vi "Read Image (MMF) (SubVI).vi"(0 "FPGA REF (MWT) IN":T3, 1 "Experiment Mode":T1=enum."Replay", 3 "Image Size":T4 {"Width" step=8; "Height" step=8}, 12 "Frame Number":u64, 13 "TimeStamp":u64) -> (4 "Image Data":T2, 6 "Data Valid?":bool)   [LabVIEW 2020]
uses:
  Controls (HOST)/Image Size.ctl
  Controls (HOST)/FPGA REF (MWT).ctl
  Controls (HOST)/Data to Disk Bundle.ctl
  Controls (HOST)/Experiment Mode.ctl
  <vilib>/Utility/error.llb/Error Cluster From Error Code.vi
  <vilib>/rvi/errors/niLvFpgaAdjustHostInterfaceError.vi
  <vilib>/rvi/interface/nirviMethod/nirviMethod.xnode
  <vilib>/rvi/errors/niLvFpgaMergeErrorWithErrorCode.vi
  <vilib>/FPGAPlugInAG/Dynamic/niLvFpga_AcquireReadRegionFifo_Dynamic.vi
  <vilib>/FPGAPlugInAG/Dynamic/niLvFpga_ReadFifo_Dynamic.vi
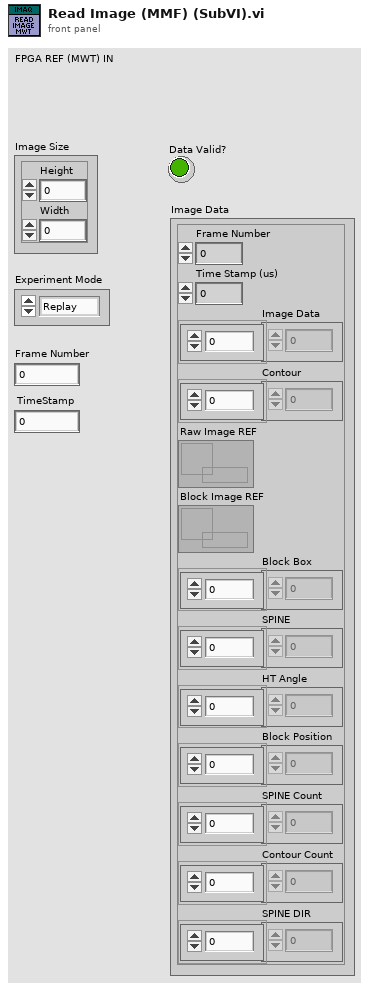
[diagram p1: front panel]
types:
  T1 = typedef "Experiment Mode.ctl" = enum16{"Live", "Replay"}
  T2 = typedef "Data to Disk Bundle.ctl" = cluster{"Frame Number":u64, "Time Stamp (us)":u64, "Image Data":u64[], "Contour":u32[], "Raw Image REF":refnum<data-value>, "Block Image REF":refnum<data-value>, "Block Box":u64[], "SPINE":u32[], "HT Angle":u64[], "Block Position":u64[], "SPINE Count":u32[], "Contour Count":u32[], "SPINE DIR":u8[]}
  T3 = typedef "FPGA REF (MWT).ctl" = refnum<k20>
  T4 = typedef "Image Size.ctl" = cluster{"Height":u16, "Width":u16}
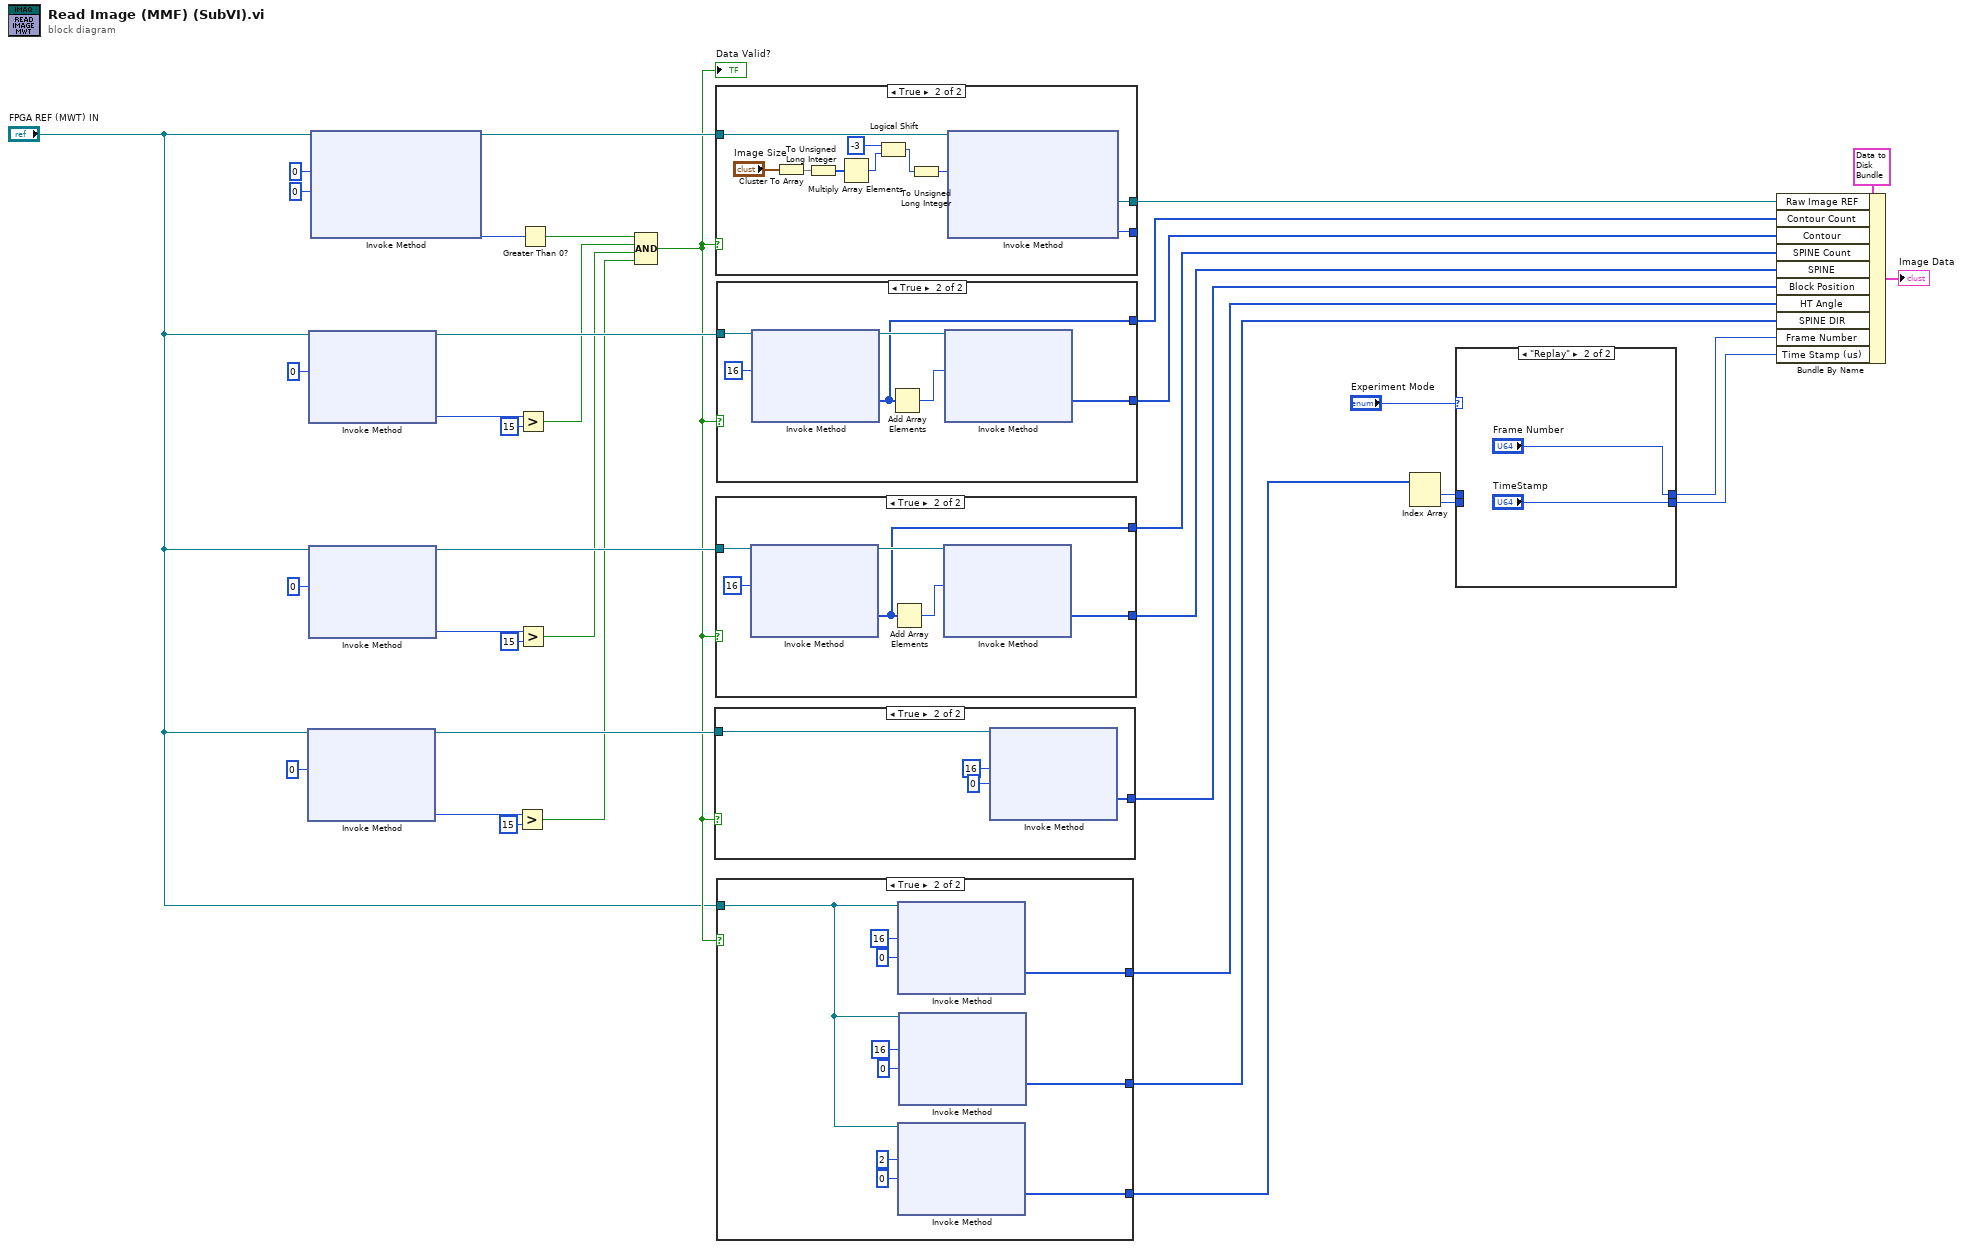
[diagram p0: block diagram]
diagram:
  n1 = xnode "Invoke Method"("FPGA VI Reference In"="FPGA REF (MWT) IN", "Number of Elements"=u32 0) -> ("FPGA VI Reference Out"=w22:T3, "Elements Remaining"=w21:u32)  [unwired: 2 in, 2 out]
  n2 = xnode "Invoke Method"("FPGA VI Reference In"="FPGA REF (MWT) IN", "Number of Elements"=u32 0) -> ("FPGA VI Reference Out"=w30:T3, "Elements Remaining"=w29:u32)  [unwired: 2 in, 2 out]
  n3 = xnode "Invoke Method"("FPGA VI Reference In"="FPGA REF (MWT) IN", "Number of Elements"=u32 0) -> ("FPGA VI Reference Out"=w23:T3, "Elements Remaining"=w24:u32)  [unwired: 2 in, 2 out]
  n4 = xnode "Invoke Method"("FPGA VI Reference In"="FPGA REF (MWT) IN", "Number of Elements"=u32 0, "Timeout (ms)"=0) -> ("FPGA VI Reference Out"=w32:T3, "Elements Remaining"=w34:u32)  [unwired: 1 in, 3 out]
  n5 = Greater?(x=w21, y=u32 15 ("x")) -> (0:w16:bool)
  n6 = Greater?(x=w29, y=u32 15 ("x")) -> (0:w18:bool)
  n7 = Greater?(x=w24, y=u32 15 ("x")) -> (0:w17:bool)
  n8 = Greater Than 0?(x=w34) -> (x > 0?=w31:bool)
  n9 = Compound Arithmetic op=AND(w31, w18, w17, w16) -> (w10:bool)
  "Data Valid?" <- w10
  n10 = case shown="True" w10 {
    tunnel: w22 -> [_ w41]
    tunnel: [_ w40] -> w15
    frame False {
    }
    frame True {
      n11 = xnode "Invoke Method"("FPGA VI Reference In"=w41, "Number of Elements"=u32 16, "Timeout (ms)"=0) -> ("Data"=w40:u64[])  [unwired: 1 in, 3 out]
    }
  }
  n12 = case shown="True" w10 {
    tunnel: [_ w52] -> w36
    tunnel: w32 -> [_ w51]
    tunnel: [_ w43] -> _
    frame False {
    }
    frame True {
      n13 = Cluster To Array(cluster="Image Size") -> (array=w45:u16[])
      n14 = To Unsigned Long Integer(number=w45) -> (unsigned 32bit integer=w47:u32[])
      n15 = Multiply Array Elements(1:w47) -> (0:w50:u32)
      n16 = Logical Shift(y=i16 -3, x=w50) -> (x << y=w48:u32)
      n17 = To Unsigned Long Integer(number=w48) -> (unsigned 32bit integer=w44:u32)
      n18 = xnode "Invoke Method"("FPGA VI Reference In"=w51, "Number of Elements"=w44) -> ("Read Region Reference"=w52:refnum<data-value>, "Elements Remaining"=w43:u32)  [unwired: 2 in, 3 out]
    }
  }
  n19 = case shown="True" w10 {
    tunnel: w23 -> [_ w57]
    tunnel: [_ w55] -> w14
    tunnel: [_ w53] -> w11
    frame False {
    }
    frame True {
      n20 = xnode "Invoke Method"("FPGA VI Reference In"=w57, "Number of Elements"=u32 16) -> ("FPGA VI Reference Out"=w56:T3, "Data"=w53:u32[])  [unwired: 2 in, 2 out]
      n21 = Add Array Elements(numeric array=w53) -> (sum=w54:u32)
      n22 = xnode "Invoke Method"("FPGA VI Reference In"=w56, "Number of Elements"=w54) -> ("Data"=w55:u32[])  [unwired: 2 in, 3 out]
    }
  }
  n23 = case shown="True" w10 {
    tunnel: w30 -> [_ w63]
    tunnel: [_ w61] -> w13
    tunnel: [_ w60] -> w12
    frame False {
    }
    frame True {
      n24 = xnode "Invoke Method"("FPGA VI Reference In"=w63, "Number of Elements"=u32 16) -> ("FPGA VI Reference Out"=w62:T3, "Data"=w60:u32[])  [unwired: 2 in, 2 out]
      n25 = Add Array Elements(numeric array=w60) -> (sum=w59:u32)
      n26 = xnode "Invoke Method"("FPGA VI Reference In"=w62, "Number of Elements"=w59) -> ("Data"=w61:u32[])  [unwired: 2 in, 3 out]
    }
  }
  n27 = case shown="True" w10 {
    tunnel: "FPGA REF (MWT) IN" -> [_ w66]
    tunnel: [_ w73] -> w8
    tunnel: [_ w70] -> w7
    tunnel: [_ w65] -> w6
    frame False {
    }
    frame True {
      n28 = xnode "Invoke Method"("FPGA VI Reference In"=w66, "Number of Elements"=u32 16, "Timeout (ms)"=0) -> ("Data"=w73:u64[])  [unwired: 1 in, 3 out]
      n29 = xnode "Invoke Method"("FPGA VI Reference In"=w66, "Number of Elements"=u32 2, "Timeout (ms)"=0) -> ("Data"=w65:u64[])  [unwired: 1 in, 3 out]
      n30 = xnode "Invoke Method"("FPGA VI Reference In"=w66, "Number of Elements"=u32 16, "Timeout (ms)"=0) -> ("Data"=w70:u8[])  [unwired: 1 in, 3 out]
    }
  }
  n31 = Index Array(array=w6) -> (element #1=w2:u64, element #2=w4:u64)  [unwired: 2 in]
  n32 = case shown="\"Replay\"" "Experiment Mode" {
    tunnel: [w76 "TimeStamp"] -> w3
    tunnel: w4 -> [w76 _]
    tunnel: w2 -> [w75 _]
    tunnel: [w75 "Frame Number"] -> w1
    frame "Live", Default {
    }
    frame "Replay" {
    }
  }
  n33 = Bundle By Name(cluster=T2 {"Frame Number"=0, "Time Stamp (us)"=0, "Image Data"=[], "Contour"=[], "Raw Image REF"=refnum, "Block Image REF"=refnum, "Block Box"=[], "SPINE"=[], "HT Angle"=[], "Block Position"=[], "SPINE Count"=[], "Contour Count"=[], "SPINE DIR"=[]}, "Raw Image REF"=w36, "Contour Count"=w12, "Contour"=w13, "SPINE Count"=w11, "SPINE"=w14, "Block Position"=w15, "HT Angle"=w8, "SPINE DIR"=w7, "Frame Number"=w1, "Time Stamp (us)"=w3) -> (→"Image Data":T2)
